vi "RSZVB Load Ground Loop Circuit Model Data.vi"(7 "File Name (\"\")":string, 8 "error in (no error)":errorcluster {"code" format="%.0x"}, 9 "Function Type (0)":i32(ring) items=["Deembedding", "Embedding"], 10 "Channel (1)":i32=1, 11 "VISA session":refnum<visa-resource-name>) -> (0 "error out":errorcluster {"code" format="%.0x"}, 3 "dup VISA session":refnum<visa-resource-name>)   [LabVIEW 2011]
doc: "This VI loads data from a specified one-port (*.s1p) Touchstone file defining the characteristics of the current embedded/deembedded ground loop circuit model. The ground loop circuit model involving file import (FIMPort) must be selected before using this VI. \n\nRemote-control command(s):\nMMEMory:LOAD:VNETworks<Ch>:GLOop:DEEMbedding<Ph_pt> '<file_name>'\nMMEMory:LOAD:VNETworks<Ch>:GLOop:EMBedding<Ph_pt> '<file_name>'"
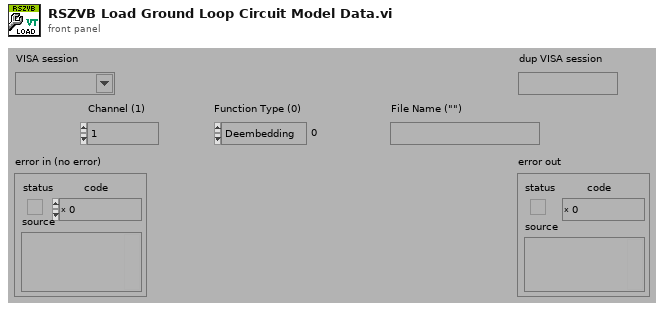
[diagram p1: front panel]
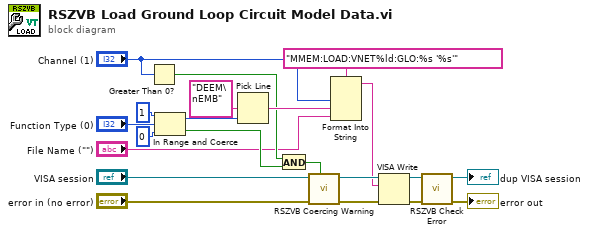
[diagram p0: block diagram]
diagram:
  n1 = Greater Than 0?(x="Channel (1)") -> (x > 0?=w10:bool)
  n2 = In Range and Coerce(upper limit=1, x="Function Type (0)", lower limit=0) -> (coerced(x)=w14:i32, In Range?=w8:bool)
  n3 = Pick Line(multi-line string="DEEM\nEMB", line index=w14) -> (output string=w11:string)  [unwired: 1 in]
  n4 = And(x=w10, y=w8) -> (x .and. y?=w9:bool)
  n5 = call "RSZVB Coercing Warning.vi"("In Range?"=w9, "error in (no error)"="error in (no error)", "VISA session"="VISA session") -> ("error out"=w17:errorcluster, "dup VISA session"=w18:refnum<visa-resource-name>)  [unwired: 7 in]
  n6 = Format Into String(format string="MMEM:LOAD:VNET%ld:GLO:%s '%s'", "Channel (1)", w11, "File Name (\"\")") -> (resulting string=w16:string)  [unwired: 2 in, 1 out]
  n7 = VISA Write(VISA resource name=w18, write buffer=w16, error in (no error)=w17) -> (VISA resource name out=w21:refnum<visa-resource-name>, error out=w20:errorcluster)  [unwired: 1 out]
  n8 = call "RSZVB Check Error.vi"("error in (no error)"=w20, "VISA session"=w21) -> ("error out"=→"error out":errorcluster, "dup VISA session"=→"dup VISA session":refnum<visa-resource-name>)  [unwired: 8 in]
